vi "Post-Install Custom Action.vi"(10 "Variant":variant) -> (0 "error out":errorcluster)   [LabVIEW 2024]
uses:
  <vilib>/Utility/file.llb/Write Delimited Spreadsheet (string).vi
  <vilib>/zip/NI_Unzip.lvlib
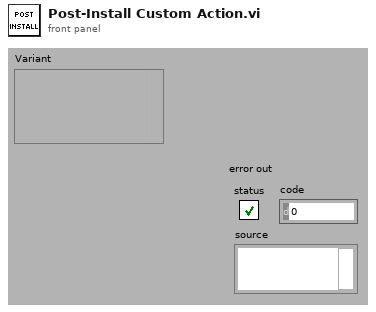
[diagram p1: front panel]
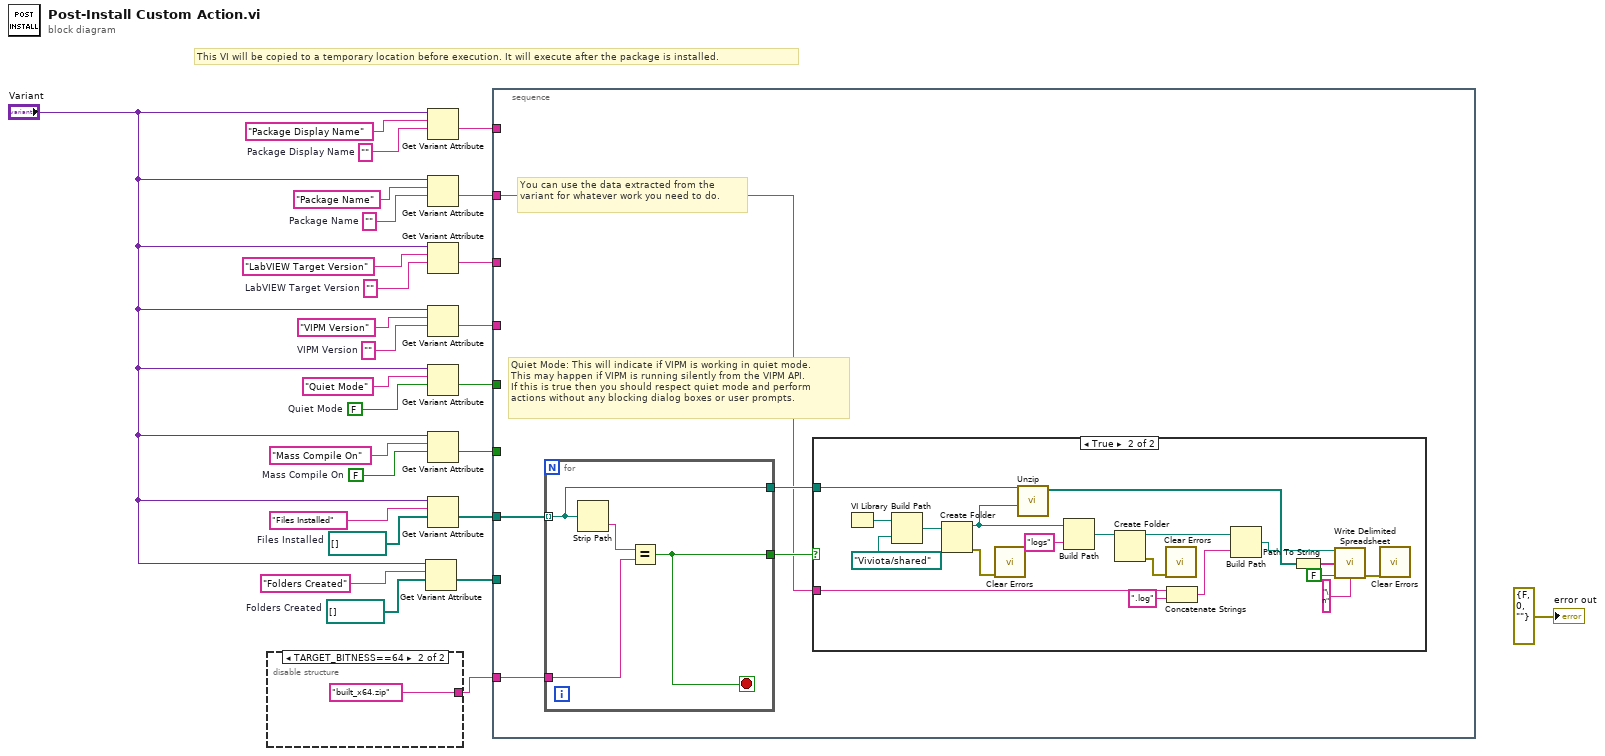
[diagram p0: block diagram]
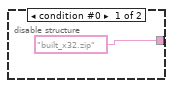
[diagram p2: hidden frame]
diagram:
  w2 = path[] []  # Folders Created
  w3 = path[] []  # Files Installed
  w9 = FALSE  # Mass Compile On
  w10 = ""  # Package Display Name
  w17 = FALSE  # Quiet Mode
  w20 = ""  # VIPM Version
  w22 = ""  # LabVIEW Target Version
  w24 = ""  # Package Name
  # "This VI will be copied to a temporary location before execution. It will execute after the package is installed."
  n1 = disable-structure shown="TARGET_BITNESS==64" {
    disable-tunnel: ["built_x32.zip" "built_x64.zip"] -> w1
    frame condition #0 {
    }
    frame condition #1 (active) {
    }
  }
  n2 = Get Variant Attribute(Variant="Variant", name="Folders Created", default value (empty Variant)=w2) -> (value=w7:path[])  [unwired: 1 in, 3 out]
  n3 = Get Variant Attribute(Variant="Variant", name="Package Display Name", default value (empty Variant)=w10) -> (value=w16:string)  [unwired: 1 in, 3 out]
  n4 = Get Variant Attribute(Variant="Variant", name="Package Name", default value (empty Variant)=w24) -> (value=w15:string)  [unwired: 1 in, 3 out]
  n5 = Get Variant Attribute(Variant="Variant", name="LabVIEW Target Version", default value (empty Variant)=w22) -> (value=w14:string)  [unwired: 1 in, 3 out]
  n6 = Get Variant Attribute(Variant="Variant", name="VIPM Version", default value (empty Variant)=w20) -> (value=w13:string)  [unwired: 1 in, 3 out]
  n7 = Get Variant Attribute(Variant="Variant", name="Quiet Mode", default value (empty Variant)=w17) -> (value=w12:bool)  [unwired: 1 in, 3 out]
  n8 = Get Variant Attribute(Variant="Variant", name="Mass Compile On", default value (empty Variant)=w9) -> (value=w11:bool)  [unwired: 1 in, 3 out]
  n9 = Get Variant Attribute(Variant="Variant", name="Files Installed", default value (empty Variant)=w3) -> (value=w6:path[])  [unwired: 1 in, 3 out]
  n10 = stacked-sequence {
    tunnel: w16 -> [_]
    tunnel: w15 -> [w30]
    tunnel: w14 -> [_]
    tunnel: w13 -> [_]
    tunnel: w12 -> [_]
    tunnel: w11 -> [_]
    tunnel: w6 -> [w32]
    tunnel: w7 -> [_]
    tunnel: w1 -> [w31]
    frame #0 {
      # "Quiet Mode: This will indicate if VIPM is working in quiet mode.\nThis may happen if VIPM is running silently from the VIPM API.\nIf this is true then you should respect quiet mode and perform\nactions without any blocking dialog boxes or user prompts."
      # "You can use the data extracted from the variant for whatever work you need to do."
      n11 = for {
        tunnel: w31 -> [w56]
        tunnel: w32 -> [w54] mode=indexing
        tunnel: [w55] -> w33
        tunnel: [w54] -> w34
        stop <- w55 stop-if-true
        n12 = Strip Path(path=w54) -> (name=w57:string)  [unwired: 1 out]
        n13 = Equal?(x=w57, y=w56) -> (x = y?=w55:bool)
      }
      n14 = case shown="True" w33 {
        tunnel: w34 -> [_ w51]
        tunnel: w30 -> [_ w44]
        frame False {
        }
        frame True {
          n15 = VI Library() -> (path=w53:path)
          n16 = Build Path(base path=w53, name or relative path=path "Viviota/shared") -> (appended path=w50:path)
          n17 = Create Folder(path (use dialog)=w50) -> (created path=w48:path, error out=w49:errorcluster)  [unwired: 2 in, 1 out]
          n18 = call <vilib>:"Clear Errors.vi"("error in (no error)"=w49) -> ()  [unwired: 5 in, 2 out]
          n19 = call <vilib>:"Unzip.vi"("Target directory (same as Zip file if empty)"=w48, "Zip file"=w51) -> ("Unzipped files"=w42:path[])  [unwired: 7 in, 2 out]
          n20 = Build Path(base path=w48, name or relative path="logs") -> (appended path=w46:path)
          n21 = Create Folder(path (use dialog)=w46) -> (created path=w40:path, error out=w45:errorcluster)  [unwired: 2 in, 1 out]
          n22 = call <vilib>:"Clear Errors.vi"("error in (no error)"=w45) -> ()  [unwired: 5 in, 2 out]
          n23 = Concatenate Strings(w44, ".log" ("string")) -> (w39:string)
          n24 = Build Path(base path=w40, name or relative path=w39) -> (appended path=w38:path)
          n25 = Path To String(path=w42) -> (string=w41:string[])
          n26 = call-poly <vilib>:"Write Delimited Spreadsheet.vi"("file path (dialog if empty)"=w38, "1D data"=w41, "append to file? (new file:F)"=FALSE, "delimiter (\\t)"="\n" ("delimiter (\\t)")) -> ("error out"=w36:errorcluster)  [unwired: 10 in, 1 out]
          n27 = call <vilib>:"Clear Errors.vi"("error in (no error)"=w36) -> ()  [unwired: 5 in, 2 out]
        }
      }
    }
  }
  "error out" <- errorcluster {"status"=FALSE, "code"=0, "source"=""} ("error out")
